vi "sub_log_fine-name.vi"(7 "Sel":enum16{"RLRobot", "RLGPS"}(ring)) -> (3 "log path":string)   [LabVIEW 2021]
uses:
  logfile-name.vi
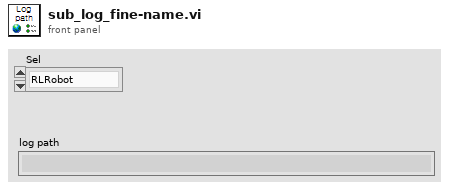
[diagram p1: front panel]
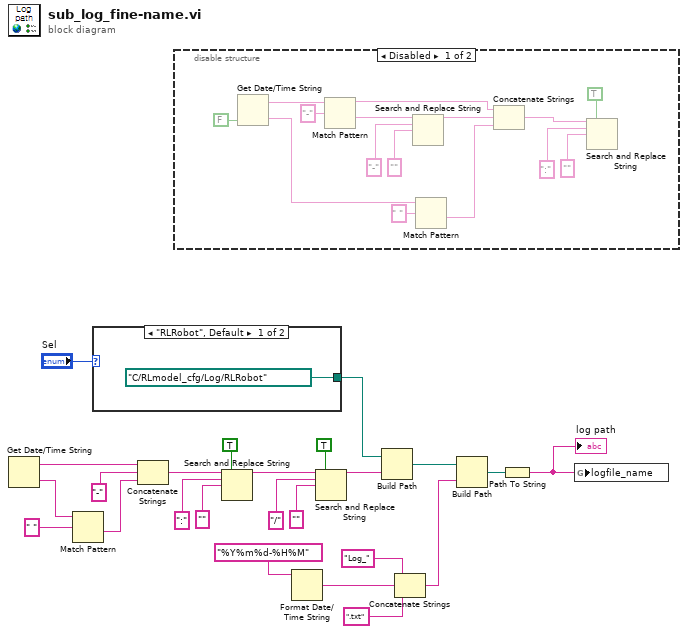
[diagram p0: block diagram]
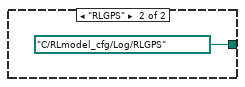
[diagram p2: hidden frame]
diagram:
  n1 = Get Date/Time String() -> (date string=w12:string, time string=w18:string)  [unwired: 3 in]
  n2 = Match Pattern(string=w18, regular expression=" " ("정규식")) -> (after substring=w17:string)  [unwired: 1 in, 3 out]
  n3 = case shown="\"RLRobot\", Default" "Sel" {
    tunnel: [path "C:/RLmodel_cfg/Log/RLRobot" ("베이스 경로") path "C:/RLmodel_cfg/Log/RLGPS" ("베이스 경로")] -> w20
    frame "RLRobot", Default {
    }
    frame "RLGPS" {
    }
  }
  n4 = Concatenate Strings(w12, "-" ("정규식"), w17) -> (w13:string)
  n5 = disable-structure shown="Disabled" {
    frame Disabled {
      n6 = Get Date/Time String(want seconds? (F)=FALSE ("초 보이기? (거짓)")) -> (date string=w36:string, time string=w33:string)  [unwired: 2 in]
      n7 = Match Pattern(string=w36, regular expression="-" ("정규식")) -> (before substring=w27:string, after substring=w31:string)  [unwired: 1 in, 2 out]
      n8 = Search and Replace String(input string=w31, search string="-" ("검색 문자열"), replace string="" ("대체 문자열(\"\")")) -> (result string=w28:string)  [unwired: 5 in, 3 out]
      n9 = Match Pattern(string=w33, regular expression=" " ("정규식")) -> (after substring=w32:string)  [unwired: 1 in, 3 out]
      n10 = Concatenate Strings(w27, w28, w32) -> (w41:string)
      n11 = Search and Replace String(replace all?=TRUE ("모두 대체? (거짓)"), input string=w41, search string=":" ("검색 문자열"), replace string="" ("대체 문자열(\"\")")) -> ()  [unwired: 4 in, 4 out]
    }
    frame Enabled {
    }
  }
  n12 = Search and Replace String(replace all?=TRUE ("모두 대체? (거짓)"), input string=w13, search string=":" ("검색 문자열"), replace string="" ("대체 문자열(\"\")")) -> (result string=w3:string)  [unwired: 4 in, 3 out]
  n13 = Format Date/Time String(time format string (%c)="%Y%m%d-%H%M") -> (date/time string=w21:string)  [unwired: 2 in]
  n14 = Search and Replace String(replace all?=TRUE ("모두 대체? (거짓)"), input string=w3, search string="/" ("검색 문자열"), replace string="" ("대체 문자열(\"\")")) -> (result string=w2:string)  [unwired: 4 in, 3 out]
  n15 = Build Path(base path=w20, name or relative path=w2) -> (appended path=w9:path)
  n16 = Concatenate Strings("Log_", w21, ".txt" ("문자열")) -> (w10:string)
  n17 = Build Path(base path=w9, name or relative path=w10) -> (appended path=w8:path)
  n18 = Path To String(path=w8) -> (string=w7:string)
  "log path" <- w7
  n19 = global write "logfile-name.vi" "logfile_name"(w7) -> ()
